vi "Pull_Slice.vi"(9 "X Values":dbl[](array[numeric]), 10 "Fit Parameters":dbl[](array[numeric]), 11 "ROI Image":sgl[][](array[numeric])) -> (0 "Constant X Slice":cluster{"X Values":dbl[], sgl[]}, 3 "Constant Y Slice":cluster{"X Values":dbl[], sgl[]})   [LabVIEW 2014]
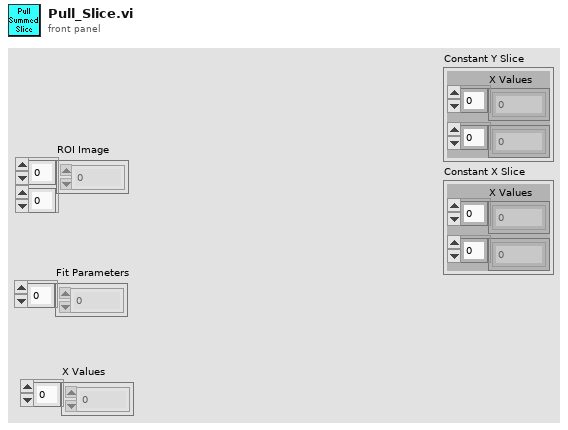
[diagram p1: front panel]
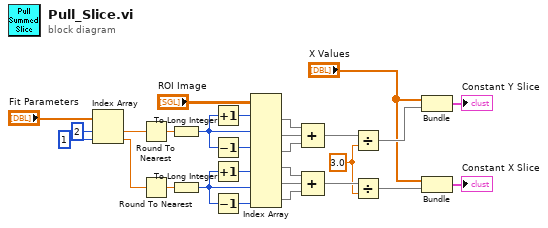
[diagram p0: block diagram]
diagram:
  w8 = sgl 3.0
  n1 = Index Array(array="Fit Parameters", index #1=2 ("index"), index #2=1 ("index")) -> (element #1=w26:dbl, element #2=w14:dbl)
  n2 = Round To Nearest(number=w26) -> (nearest integer value=w25:dbl)
  n3 = Round To Nearest(number=w14) -> (nearest integer value=w18:dbl)
  n4 = To Long Integer(number=w25) -> (32bit integer=w24:i32)
  n5 = To Long Integer(number=w18) -> (32bit integer=w17:i32)
  n6 = Increment(x=w24) -> (x+1=w22:i32)
  n7 = Decrement(x=w24) -> (x-1=w23:i32)
  n8 = Increment(x=w17) -> (x+1=w16:i32)
  n9 = Decrement(x=w17) -> (x-1=w15:i32)
  n10 = Index Array(array="ROI Image", index (row) #1=w22, index (row) #2=w24, index (row) #3=w23, index (col) #4=w16, index (col) #5=w17, index (col) #6=w15) -> (element #1=w21:sgl[], element #2=w20:sgl[], element #3=w19:sgl[], element #4=w12:sgl[], element #5=w13:sgl[], element #6=w11:sgl[])  [unwired: 6 in]
  n11 = Compound Arithmetic op=ADD(w21, w20, w19) -> (w10:sgl[])
  n12 = Compound Arithmetic op=ADD(w12, w13, w11) -> (w9:sgl[])
  n13 = Divide(x=w10, y=w8) -> (x/y=w7:sgl[])
  n14 = Divide(x=w9, y=w8) -> (x/y=w6:sgl[])
  n15 = Bundle("X Values"="X Values", w7) -> (→"Constant Y Slice":cluster{"X Values":dbl[], sgl[]})  [unwired: 1 in]
  n16 = Bundle("X Values"="X Values", w6) -> (→"Constant X Slice":cluster{"X Values":dbl[], sgl[]})  [unwired: 1 in]
